vi "Register.vi"(7 "Event":refnum<class "Event.lvclass">, 8 "Error In":errorcluster, 9 "Sink Event Fire Handler":refnum<class "Event Generated Msg.lvclass">, 10 "Registrant Details":T1, 11 "Event Source In":refnum<class "Event Source.lvclass">) -> (0 "Error Out":errorcluster, 3 "Event Source Out":refnum<class "Event Source.lvclass">)   [LabVIEW 2016, in "Event Source.lvlib" / "Event Source.lvclass"]
doc: "This method registers a specific Actors Enqueuer and a Zero Coupling based message (inheriting from Event Generated Msg.lvclass) to used when the specified Event is Fired anywhere inside the Event Source Actor."
uses:
  Event Source.lvclass
  Event/Event.lvclass
  Sink Details.ctl
  <vilib>/ActorFramework/Message Enqueuer/Message Enqueuer.lvclass
  Event Source Messages/Event Generated Msg/Event Generated Msg.lvclass
  Event Source.lvclass/Event Source.ctl
  Event Handler Details.ctl
  Event/Event.lvclass/Event.ctl
  <vilib>/Utility/error.llb/Error Cluster From Error Code.vi
  <resource>/AFDebug/Localized Strings.vi
  <resource>/AFDebug/Get Clone Name.vi
  <resource>/AFDebug/Actor Registry.vi
  <resource>/AFDebug/TDM Registry.vi
  <vilib>/ErrorRing/Error Ring.xnode
  <resource>/AFDebug/AF Debug.lvlib
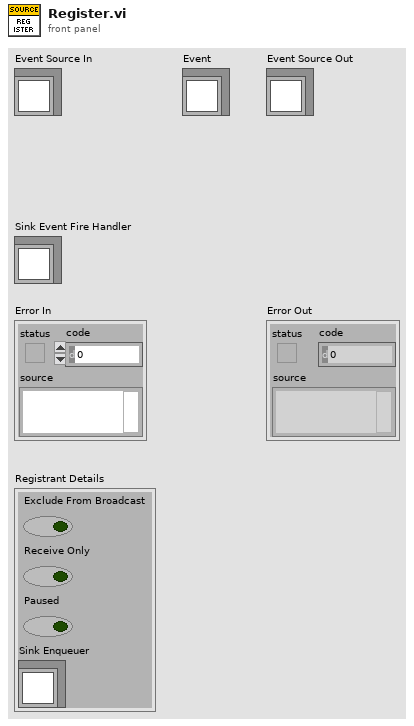
[diagram p1: front panel]
types:
  T1 = typedef "Event Source.lvlib/Event Source.lvclass/Sink Details.ctl" = cluster{"Exclude From Broadcast":bool, "Receive Only":bool, "Paused":bool, "Sink Enqueuer":refnum<class "Message Enqueuer.lvclass">}
  T2 = typedef "Event Source.lvlib/Event Source.lvclass/Event Handler Details.ctl" = cluster{"Exclude From Broadcast":bool, "Paused":bool, "Sink Event Fire Handler":refnum<class "Event Generated Msg.lvclass">}
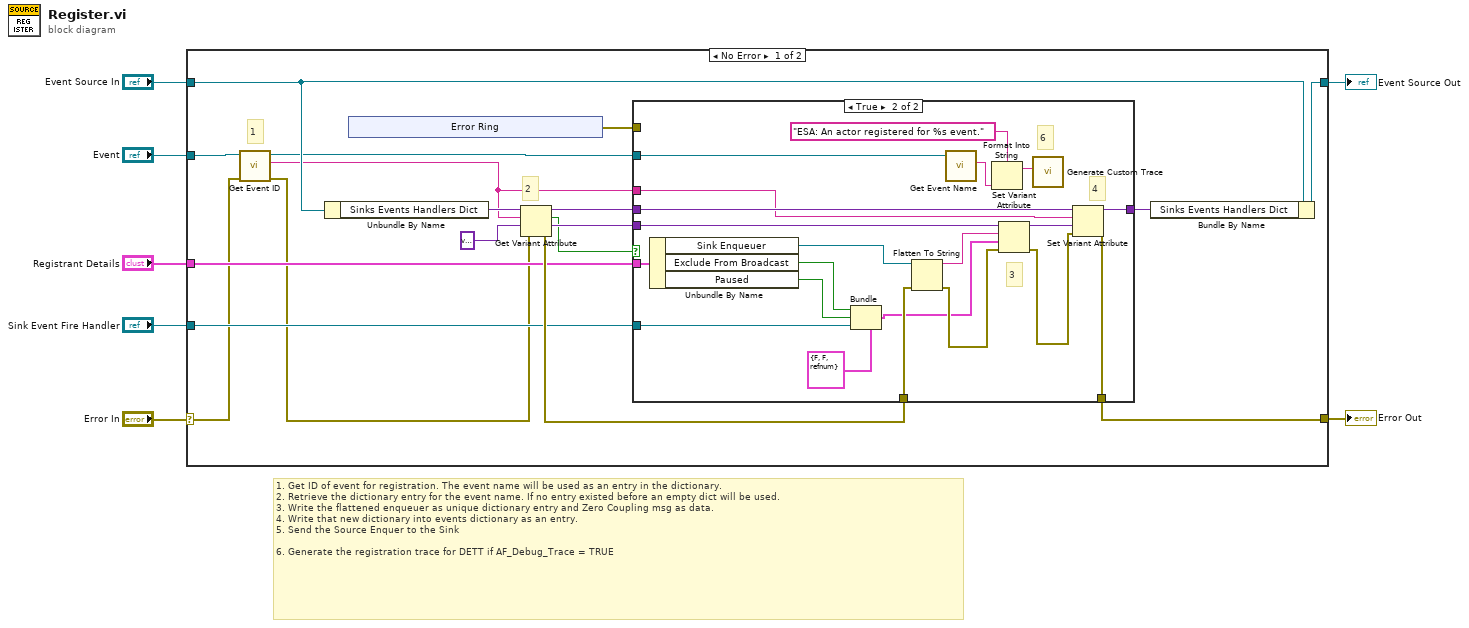
[diagram p0: block diagram]
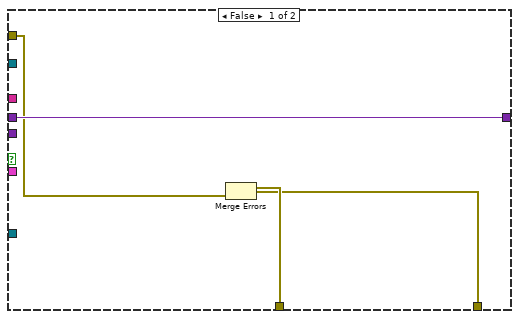
[diagram p2: hidden frame]
diagram:
  # "1. Get ID of event for registration. The event name will be used as an entry in the dictionary.\n2. Retrieve the dictionary entry for the event name. If no entry existed before an empty dict will be used.\n3. Write the flattened enqueuer as unique dictionary entry and Zero Coupling msg as data.\n4. Write that new dictionary into events dictionary as an entry.\n5. Send the Source Enquer to the Sink \n\n6. Generate the registration trace for DETT if AF_Debug_Trace = TRUE"
  n1 = case shown="No Error" "Error In" {
    selector: "Error In" -> [w13 w55]
    tunnel: "Event Source In" -> [w15 w56]
    tunnel: "Event" -> [w14 _]
    tunnel: [w21 w56] -> w6
    tunnel: [w25 w55] -> w4
    tunnel: "Registrant Details" -> [w16 _]
    tunnel: "Sink Event Fire Handler" -> [w20 _]
    frame No Error {
      # "2"
      # "1"
      n2 = call-dynamic "Get Event ID.vi"("error in (no error)"=w13, "Event in"=w14) -> ("error out"=w11:errorcluster, "Event ID"=w12:string, "Event out"=w9:refnum<class "Event.lvclass">)  [unwired: 7 in]
      n3 = Unbundle By Name(w15) -> ("Sinks Events Handlers Dict"=w24:variant)
      n4 = xnode "Error Ring"() -> ("error out"=w8:errorcluster)
      n5 = Get Variant Attribute(Variant=w24, name=w12, default value (empty Variant)=variant ("variant"), error in=w11) -> (duplicate Variant=w23:variant, found=w10:bool, value=w18:variant, error out=w22:errorcluster)
      n6 = case shown="True" w10 {
        tunnel: [w32 w54] -> w25
        tunnel: w23 -> [w31 w53]
        tunnel: w22 -> [w33 w52]
        tunnel: w20 -> [_ w35]
        tunnel: [w31 w49] -> w19
        tunnel: w18 -> [_ w48]
        tunnel: w16 -> [_ w40]
        tunnel: w12 -> [_ w47]
        tunnel: w9 -> [_ w41]
        tunnel: w8 -> [w30 _]
        frame False {
          n7 = Merge Errors(w33, w30) -> (w32:errorcluster)
        }
        frame True {
          # "6"
          # "4"
          # "3"
          n8 = Unbundle By Name(w40) -> ("Sink Enqueuer"=w39:refnum<class "Message Enqueuer.lvclass">, "Exclude From Broadcast"=w37:bool, "Paused"=w36:bool)
          n9 = Bundle(cluster=T2 {"Exclude From Broadcast"=FALSE, "Paused"=FALSE, "Sink Event Fire Handler"=refnum} ("Sink Settings"), "Exclude From Broadcast"=w37, "Paused"=w36, "Sink Event Fire Handler"=w35) -> (w34:T2)
          n10 = Flatten To String(anything=w39, error in (no error)=w52) -> (data string=w51:string, error out=w46:errorcluster)  [unwired: 2 in, 1 out]
          n11 = call "Get Event Name.vi"("Event In"=w41) -> ("Name"=w42:string)  [unwired: 9 in, 1 out]
          n12 = Format Into String(format string="ESA: An actor registered for %s event." ("Custom Action"), w42) -> (resulting string=w43:string)  [unwired: 2 in, 1 out]
          n13 = Set Variant Attribute(Variant=w48, name=w51, value=w34, error in=w46) -> (Variant out=w50:variant, error out=w45:errorcluster)  [unwired: 1 out]
          n14 = call <resource>:"Generate Custom Trace.vi"("Custom Action"=w43) -> ()  [unwired: 11 in]
          n15 = Set Variant Attribute(Variant=w53, name=w47, value=w50, error in=w45) -> (Variant out=w49:variant, error out=w54:errorcluster)  [unwired: 1 out]
        }
      }
      n16 = Bundle By Name(cluster=w15, "Sinks Events Handlers Dict"=w19) -> (w21:refnum<class "Event Source.lvclass">)
    }
    frame Error {
    }
  }
  "Error Out" <- w4
  "Event Source Out" <- w6
